vi "Prep Recipe.vi"(8 "error in (no error)":errorcluster, 11 "Recipe Process in":refnum<class "Recipe Process.lvclass">) -> (0 "error out":errorcluster, 3 "Recipe Process out":refnum<class "Recipe Process.lvclass">)   [LabVIEW 2022 SP3, in "Recipe Process.lvlib" / "Recipe Process.lvclass"]
uses:
  Recipe Process.lvclass
  Recipe Process.lvclass/Recipe Process.ctl
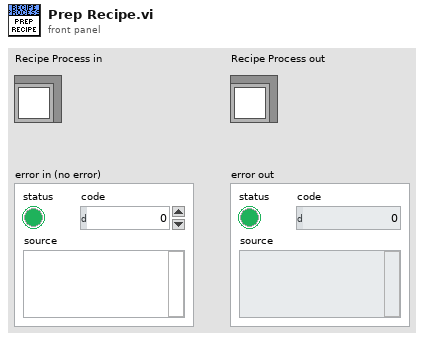
[diagram p1: front panel]
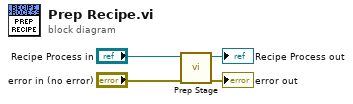
[diagram p0: block diagram]
diagram:
  n1 = call "Prep Stage.vi"("error in (no error)"="error in (no error)", "Recipe Process in"="Recipe Process in") -> ("error out"=→"error out":errorcluster, "Recipe Process out"=→"Recipe Process out":refnum<class "Recipe Process.lvclass">)  [unwired: 8 in]
